vi "fsk_test.vi"() -> ()   [LabVIEW 2012]
uses:
  <vilib>/addons/Modulation/Digital/General/MT Generate FSK System Parameters(M).vi
  <vilib>/addons/Modulation/Digital/General/MT Generate FSK Synchronization Parameters (bit array).vi
  <vilib>/addons/Modulation/niDMT.lvlib
panel:
  out "Iterations":i32
  in  "stop":bool
  out "Recovered Signal":dbl[](graph)
  out "Transmitted Signal":dbl[](graph)
  in  "samples per symbol (16)":i32=32
  out "Recovered Phase":dbl[](graph)
  out "Transmitted Phase":dbl[](graph)
  out "Recovered Magnitude":dbl[](graph)
  out "Transmitted Magnitude":dbl[](graph)
  out "appended array":i8[](array[numeric])
  out "ber":dbl
  out "error out":errorcluster
  out "output bit stream":i8[](array[numeric])
  out "Key Bit Sequence":i8[](array[numeric])
  in  "Packet Length":i32=100
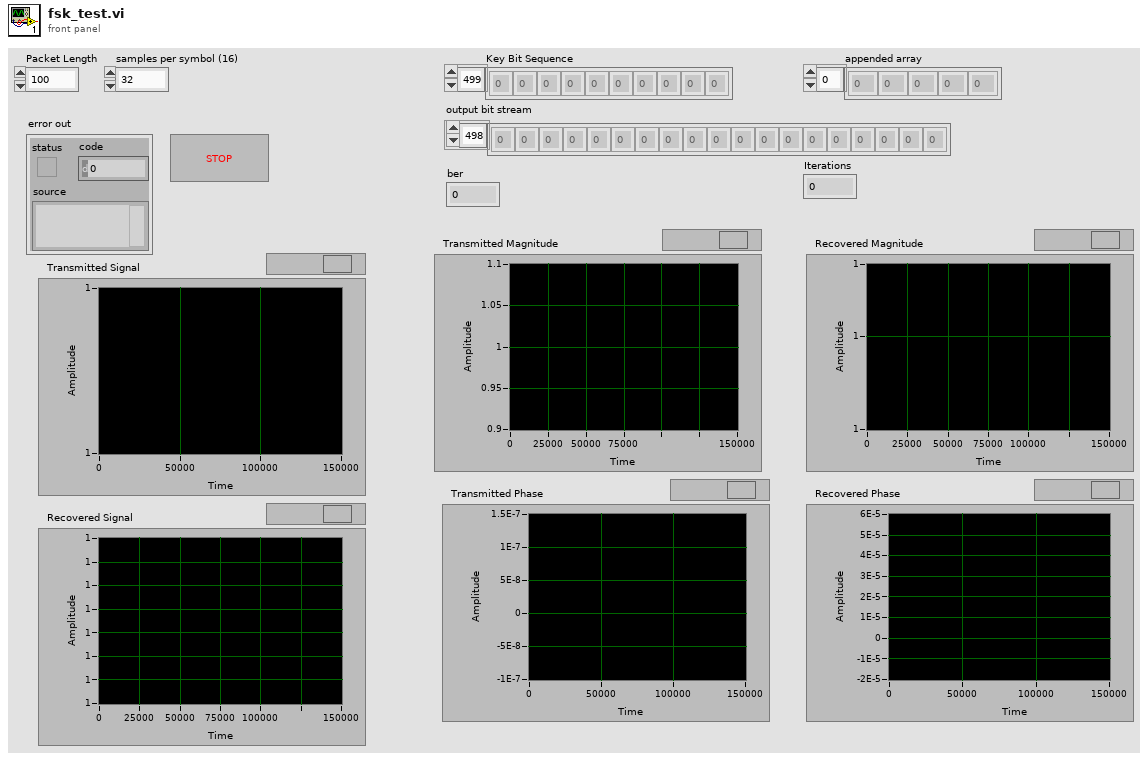
[diagram p1: front panel]
types:
  T1 = enum16{"FSK", "PSK", "QAM", "MSK", "PAM", "ASK", "CPM"}
  T2 = cluster{"samples per symbol (16)":i32, "symbol map":dbl[], "symbol phase continuity":enum16{"continuous", "discontinuous"}}
  T3 = typedef "niAMT.lvlib/Complex Data Waveform.ctl" = cluster{"t0":dbl, "dt":dbl, "Y":cdb[]}
  T4 = cluster{"expected sync location (symbols)":i32, "sync sequence":cdb[], "sync location uncertainty (symbols)":i32, "sync indent (symbols)":i32}
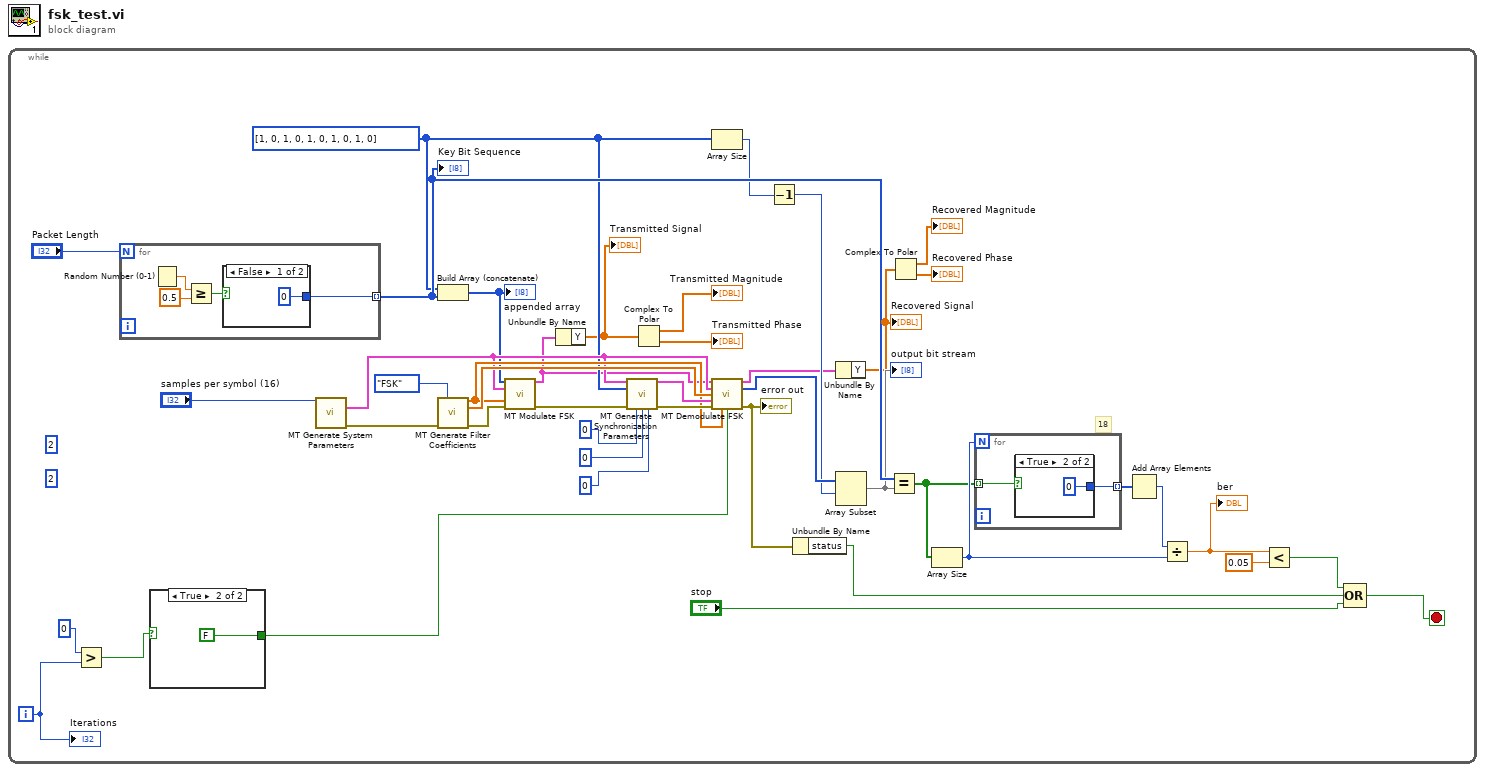
[diagram p0: block diagram]
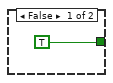
[diagram p2: hidden frame]
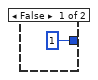
[diagram p3: hidden frame]
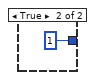
[diagram p4: hidden frame]
diagram:
  n1 = while {
    i -> [w10]
    stop <- w3 stop-if-true
    (unwired) 2
    (unwired) 2
    w21 = i8[] [1, 0, 1, 0, 1, 0, 1, 0, 1, 0] ("sync bits")
    # "18"
    n2 = Greater?(x=0, y=w10) -> (0:w8:bool)
    n3 = for {
      N: "Packet Length" -> [_]
      tunnel: [w51] -> w26 mode=indexing
      n4 = Random Number (0-1)() -> (number: 0 to 1=w53:dbl)
      n5 = Greater Or Equal?(x=w53, y=0.5) -> (x >= y?=w52:bool)
      n6 = case shown="False" w52 {
        tunnel: [i8 0 i8 1] -> w51
        frame False {
        }
        frame True {
        }
      }
    }
    "Key Bit Sequence" <- w26
    n7 = case shown="True" w8 {
      tunnel: [TRUE FALSE] -> w7
      frame False {
      }
      frame True {
      }
    }
    n8 = call-poly <vilib>:"MT Generate System Parameters.vi"("samples per symbol (16)"="samples per symbol (16)") -> ("FSK system parameters"=w35:T2, "error out"=w43:errorcluster)  [unwired: 12 in, 1 out]
    n9 = Build Array (concatenate)(w21, w26) -> (w34:i8[])
    "appended array" <- w34
    n10 = call <vilib>:"MT Generate Filter Coefficients.vi"("modulation type"=T1."FSK", "error in (no error)"=w43) -> ("pulse shaping filter coefficients"=w37:dbl[], "matched filter coefficients"=w39:dbl[], "error out"=w42:errorcluster)  [unwired: 11 in]
    n11 = call <vilib>:"MT Modulate FSK.vi"("input bit stream"=w34, "FSK system parameters"=w35, "pulse shaping filter coefficients"=w37, "error in (no error)"=w42) -> ("output complex waveform"=w18:T3, "error out"=w41:errorcluster)  [unwired: 9 in, 1 out]
    n12 = Unbundle By Name(w18) -> ("Y"=w13:cdb[])
    "Transmitted Signal" <- w13
    n13 = call-poly <vilib>:"MT Generate Synchronization Parameters.vi"("FSK system parameters"=w35, "sync bits"=w21, "error in (no error)"=w41, "expected sync location (symbols)"=0, "sync location uncertainty (symbols)"=0, "sync indent (symbols)"=0) -> ("FSK synchronization parameters"=w38:T4, "error out"=w40:errorcluster)  [unwired: 8 in]
    n14 = Complex To Polar(r * e^(i*theta)=w13) -> (r=→"Transmitted Magnitude":dbl[], theta=→"Transmitted Phase":dbl[])
    n15 = Array Size(array=w21) -> (size(s)=w23:i32)
    n16 = call <vilib>:"MT Demodulate FSK.vi"("input complex waveform"=w18, "FSK system parameters"=w35, "matched filter coefficients"=w39, "synchronization parameters"=w38, "error in (no error)"=w40, "pulse shaping filter coefficients"=w37, "reset? (T)"=w7) -> ("recovered complex waveform"=w17:T3, "output bit stream"=w25:i8[], "error out"=w11:errorcluster)  [unwired: 4 in, 2 out]
    "error out" <- w11
    n17 = Decrement(x=w23) -> (x-1=w22:i32)
    n18 = Unbundle By Name(w11) -> ("status"=w5:bool)
    n19 = Unbundle By Name(w17) -> ("Y"=w12:cdb[])
    "Recovered Signal" <- w12
    n20 = Array Subset(array=w25, index=w22) -> (w24:i8[])  [unwired: 1 in]
    "output bit stream" <- w24
    n21 = Equal?(x=w26, y=w24) -> (x = y?=w27:bool[])
    n22 = Complex To Polar(r * e^(i*theta)=w12) -> (r=→"Recovered Magnitude":dbl[], theta=→"Recovered Phase":dbl[])
    n23 = Array Size(array=w27) -> (size(s)=w28:i32)
    n24 = for {
      N: w28 -> [_]
      tunnel: [w48] -> w30 mode=indexing
      tunnel: w27 -> [w47] mode=indexing
      n25 = case shown="True" w47 {
        tunnel: [1 0] -> w48
        frame False {
        }
        frame True {
        }
      }
    }
    n26 = Add Array Elements(numeric array=w30) -> (sum=w29:i32)
    n27 = Divide(x=w29, y=w28) -> (x/y=w2:dbl)
    "ber" <- w2
    n28 = Less?(x=w2, y=0.05) -> (x < y?=w6:bool)
    n29 = Compound Arithmetic op=OR(w6, w5, "stop") -> (w3:bool)
    "Iterations" <- w10
  }
